vi "Sequence.InitializeMain.vi"(8 "error in (no error)":errorcluster, 9 "IterationInfo":T4, 10 "Steps":T1[](array[typedef]), 11 "Iterations":u32) -> (0 "error out":errorcluster, 3 "Refs":T8)   [LabVIEW 2013, in "Simple Sequence Tools - Editor.lvlib"]
uses:
  Simple Sequence Tools - Editor.lvlib
  Types/Sequence.MainSeqRefs.ctl
  NationalInstruments.VeriStand.RealTimeSequenceDefinitionApi
  Shared/Types/Channel.Properties.ctl
  Types/Compiled.StepProperties.ctl
  Types/Compiled.IOStateProperties.ctl
  Types/Compiled.StepElementProperties.ctl
  Shared/Types/Step.Types.ctl
  Types/Compiled.StepCondition.ctl
  Types/Conditions.OperationTypes.ctl
  Shared/SubVIs/Main.Constants.vi
  Shared/Simple Sequence Tools - Shared.lvlib
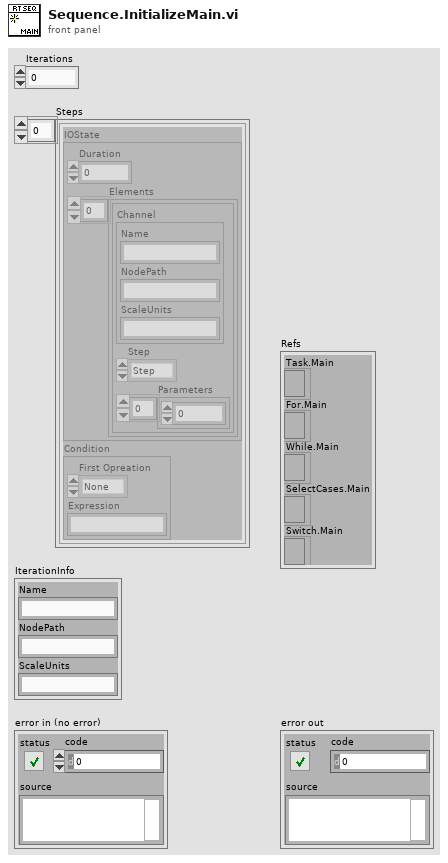
[diagram p1: front panel]
types:
  T1 = typedef "Simple Sequence Tools - Editor.lvlib/Compiled.StepProperties.ctl" = cluster{"IOState":T2, "Condition":T6}
  T2 = typedef "Simple Sequence Tools - Editor.lvlib/Compiled.IOStateProperties.ctl" = cluster{"Duration":dbl, "Elements":T3[]}
  T3 = typedef "Simple Sequence Tools - Editor.lvlib/Compiled.StepElementProperties.ctl" = cluster{"Channel":T4, "Step":T5, "Parameters":dbl[]}
  T4 = typedef "Simple Sequence Tools - Shared.lvlib/Channel.Properties.ctl" = cluster{"Name":string, "NodePath":string, "ScaleUnits":string}
  T5 = typedef "Simple Sequence Tools - Shared.lvlib/Step.Types.ctl" = enum8{"Step", "iStep", "Ramp", "Unchanged", "Unknown"}
  T6 = typedef "Simple Sequence Tools - Editor.lvlib/Compiled.StepCondition.ctl" = cluster{"First Opreation":T7, "Expression":string}
  T7 = typedef "Simple Sequence Tools - Editor.lvlib/Conditions.OperationTypes.ctl" = enum8{"None", "&&", "||"}
  T8 = typedef "Simple Sequence Tools - Editor.lvlib/Sequence.MainSeqRefs.ctl" = cluster{"Task.Main":refnum<k24>, "For.Main":refnum<k24>, "While.Main":refnum<k24>, "SelectCases.Main":refnum<k24>, "Switch.Main":refnum<k24>}
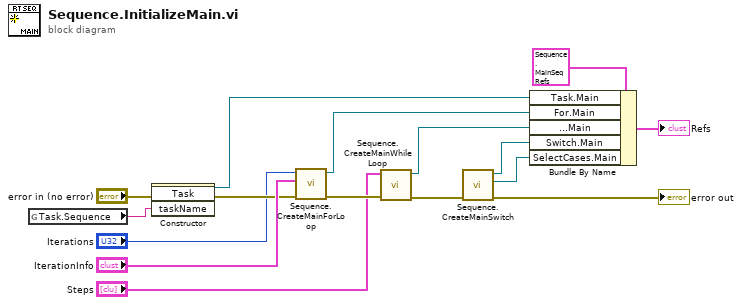
[diagram p0: block diagram]
diagram:
  n1 = global read "Main.Constants.vi" "Task.Sequence"() -> (w9:string)
  n2 = constructor class="Task"(error in="error in (no error)", "taskName"=w9) -> (reference out=w11:refnum<k24>, error out=w6:errorcluster)  [unwired: 2 in, 2 out]
  n3 = call "Sequence.CreateMainForLoop.vi"("error in (no error)"=w6, "IterationInfo"="IterationInfo", "Iterations"="Iterations") -> ("error out"=w4:errorcluster, "ForLoop Ref"=w12:refnum<k24>)  [unwired: 7 in]
  n4 = call "Sequence.CreateMainWhileLoop.vi"("error in (no error)"=w4, "Steps"="Steps") -> ("error out"=w1:errorcluster, "WhileLoop Ref"=w13:refnum<k24>)  [unwired: 8 in]
  n5 = call "Sequence.CreateMainSwitch.vi"("error in (no error)"=w1) -> ("error out"=→"error out":errorcluster, "Cases Ref"=w14:refnum<k24>, "Switch Ref"=w15:refnum<k24>)  [unwired: 8 in]
  n6 = Bundle By Name(cluster=T8 {"Task.Main"=refnum, "For.Main"=refnum, "While.Main"=refnum, "SelectCases.Main"=refnum, "Switch.Main"=refnum}, "Task.Main"=w11, "For.Main"=w12, "While.Main"=w13, "Switch.Main"=w15, "SelectCases.Main"=w14) -> (→"Refs":T8)
